vi "Enable IO PWM.vi"(8 "error in":errorcluster, 9 "State":bool, 10 "Number":u8 max=6 step=1, 11 "VISA resource name":refnum<visa-resource-name>) -> (0 "error out":errorcluster, 3 "VISA resource name out":refnum<visa-resource-name>)   [LabVIEW 2024, in "IT-M3900C.lvlib"]
doc: "This command sets IO PWM enable, the first parameter is the selected IO port serial number, the second parameter is to set IO port PWM start state.\n<b>Number</b>\n0-6\n<b>State</b>\n0:Close the State\n1:Open the state"
uses:
  IT-M3900C.lvlib
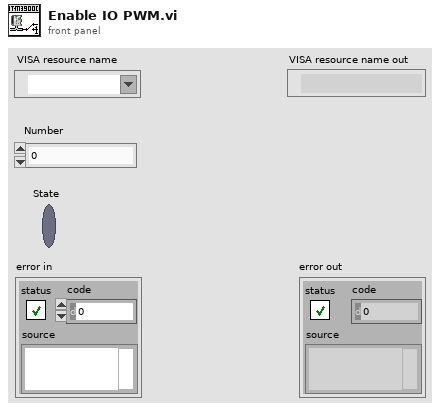
[diagram p1: front panel]
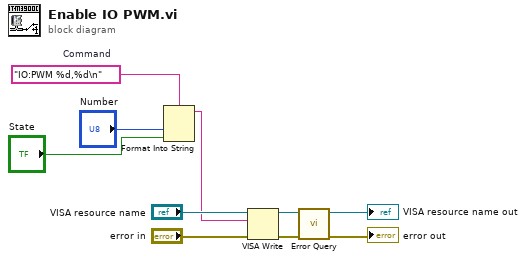
[diagram p0: block diagram]
diagram:
  w4 = "IO:PWM %d,%d\n"  # Command
  n1 = Format Into String(format string=w4, "Number", "State") -> (resulting string=w2:string)  [unwired: 2 in, 1 out]
  n2 = VISA Write(VISA resource name="VISA resource name", write buffer=w2, error in (no error)="error in") -> (VISA resource name out=w7:refnum<visa-resource-name>, error out=w8:errorcluster)  [unwired: 1 out]
  n3 = call "Error Query.vi"("error in"=w8, "VISA resource name"=w7) -> ("error out"=→"error out":errorcluster, "VISA resource name out"=→"VISA resource name out":refnum<visa-resource-name>)  [unwired: 6 in, 2 out]
